vi "Client Receive.vi"(8 "error in (no error)":errorcluster, 10 "Timeout":dbl=10.0 format="%#_13g", 11 "Telegram Class in":refnum<class "Telegram Class.lvclass">) -> (0 "error out":errorcluster, 2 "UTF-8 String Out":string, 3 "Telegram Class out":refnum<class "Telegram Class.lvclass">)   [LabVIEW 2015, in "Telegram Library.lvlib" / "Telegram Class.lvclass"]
doc: "Created IvanLis by LabVIEW Portal\nProfile: http://labviewportal.org/memberlist.php?mode=viewprofile&u=987\neMail: IvanLisanov@gMail.com\nTelegram: https://t.me/IvanLis"
uses:
  Telegram Class.lvclass
  Telegram Class.lvclass/Telegram Class.ctl
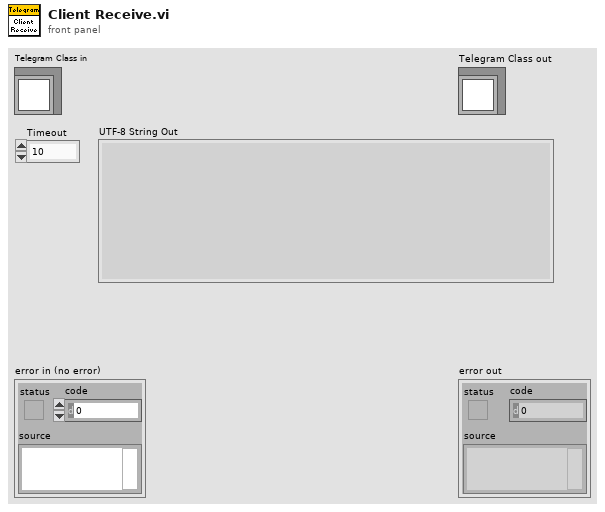
[diagram p1: front panel]
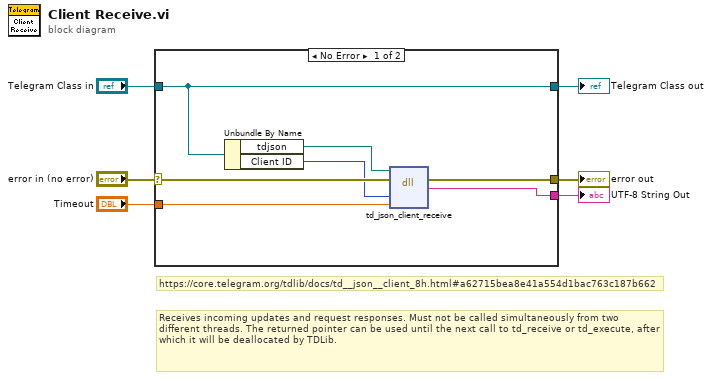
[diagram p0: block diagram]
diagram:
  # "Receives incoming updates and request responses. Must not be called simultaneously from two different threads. The returned pointer can be used until the next call to td_receive or td_execute, after which it will be deallocated by TDLib."
  # "https://core.telegram.org/tdlib/docs/td__json__client_8h.html#a62715bea8e41a554d1bac763c187b662"
  n1 = case shown="No Error" "error in (no error)" {
    selector: "error in (no error)" -> [w12 w15]
    tunnel: [w8 w15] -> w5
    tunnel: [w13 w14] -> w3
    tunnel: "Telegram Class in" -> [w13 w14]
    tunnel: "Timeout" -> [w9 _]
    tunnel: [w7 _] -> w1
    frame No Error {
      n2 = Unbundle By Name(w13) -> ("tdjson"=w11:path, "Client ID"=w10:i32)
      n3 = dll-call lib="C:/Users/Ivan/Desktop/Telegram/Project/DLL/tdjson-x32.dll" fn="td_json_client_receive"(path in=w11, error in=w12, "Client ID"=w10, "TimeOut"=w9) -> (error out=w8:errorcluster, "String"=w7:string)  [unwired: 3 in, 1 out]
    }
    frame Error {
    }
  }
  "error out" <- w5
  "Telegram Class out" <- w3
  "UTF-8 String Out" <- w1
